vi "5.2.1.-SubVI Suavizado Gaussiano.vi"(6 "Capa de color":u32[][](array[numeric]), 7 "Sigma":dbl, 9 "T":dbl) -> (1 "Array out":i32[][](array[numeric]), 2 "J":i32[][](array[numeric]), 3 "h":dbl[][](array[numeric]))   [LabVIEW 2020]
panel:
  # "Visión Artificial - Reconocimiento de Bordes - Suavizado Filtro Gaussiano\nDiego Cervantes Rodríguez\ndicer0.com"
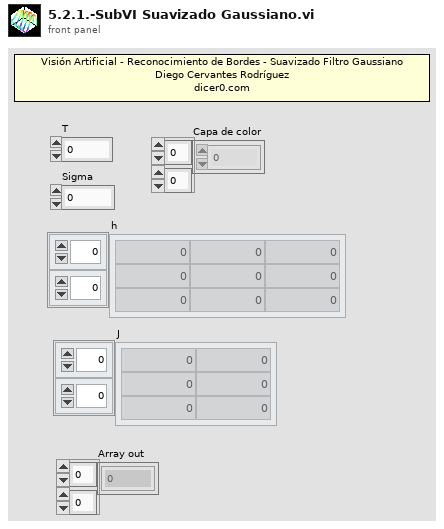
[diagram p1: front panel]
types:
  T1 = typedef "NI_Matrix.lvlib/RealMatrix.ctl" = dbl[][]
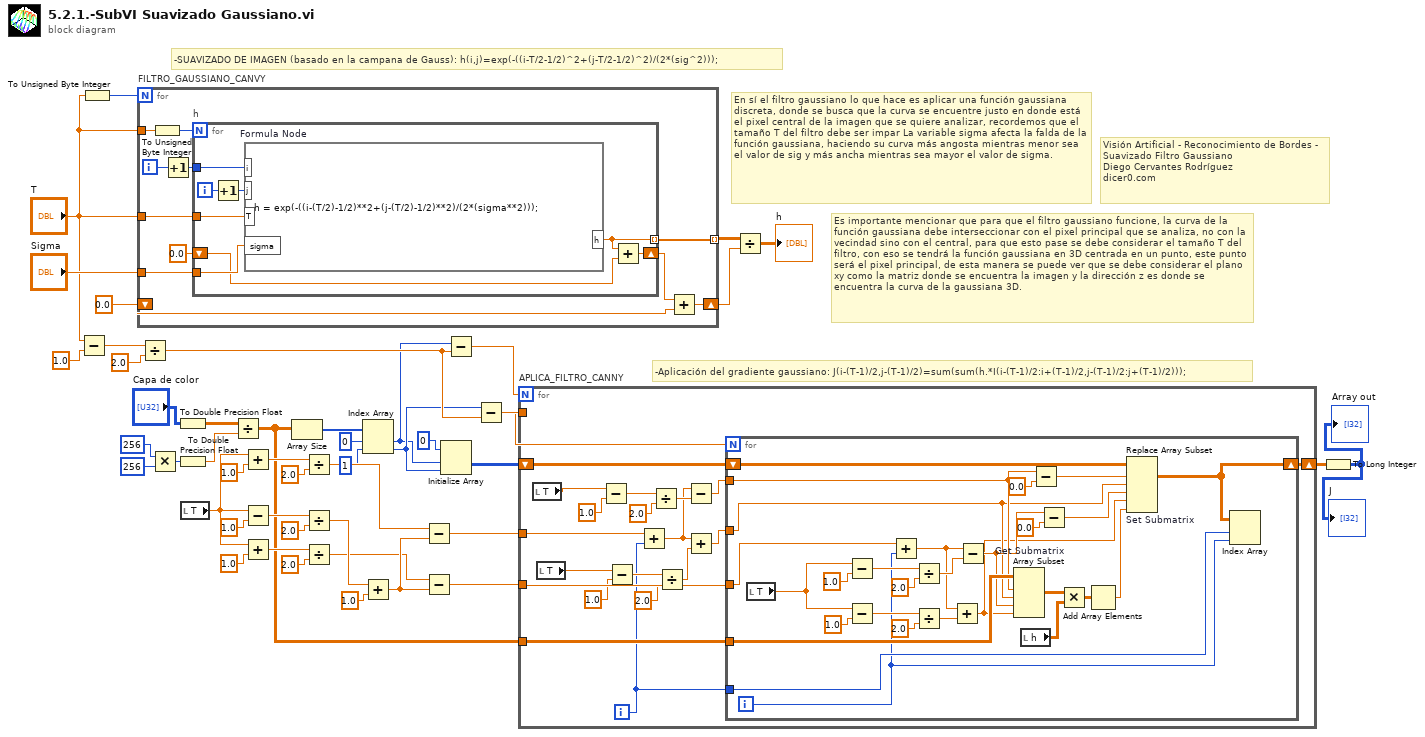
[diagram p0: block diagram]
diagram:
  # "Visión Artificial - Reconocimiento de Bordes - Suavizado Filtro Gaussiano\nDiego Cervantes Rodríguez\ndicer0.com"
  # "-Aplicación del gradiente gaussiano: J(i-(T-1)/2,j-(T-1)/2)=sum(sum(h.*I(i-(T-1)/2:i+(T-1)/2,j-(T-1)/2:j+(T-1)/2)));"
  # "Es importante mencionar que para que el filtro gaussiano funcione, la curva de la función gaussiana debe interseccionar con el pixel principal que se analiza, no con la vecindad sino con el central, para que esto pase se debe considerar el tamaño T del filtro, con eso se tendrá la función gaussiana en 3D centrada en un punto, este punto será el pixel principal, de esta manera se puede ver que se debe considerar el plano xy como la matriz donde se encuentra la imagen y la dirección z es donde se encuentra la curva de la gaussiana 3D."
  # "En sí el filtro gaussiano lo que hace es aplicar una función gaussiana discreta, donde se busca que la curva se encuentre justo en donde está el pixel central de la imagen que se quiere analizar, recordemos que el tamaño T del filtro debe ser impar La variable sigma afecta la falda de la función gaussiana, haciendo su curva más angosta mientras menor sea el valor de sig y más ancha mientras sea mayor el valor de sigma."
  # "-SUAVIZADO DE IMAGEN (basado en la campana de Gauss): h(i,j)=exp(-((i-T/2-1/2)^2+(j-T/2-1/2)^2)/(2*(sig^2)));"
  n1 = Subtract(x="T", y=1.0) -> (x-y=w20:dbl)
  n2 = To Unsigned Byte Integer(number="T") -> (unsigned 8bit integer=w9:u8)
  n3 = for "FILTRO_GAUSSIANO_CANVY" {
    N: w9 -> [_]
    tunnel: "T" -> [w47]
    tunnel: "T" -> [w57]
    tunnel: "Sigma" -> [w56]
    shift-right: [w53] -> w13
    shift-left: 0.0 ("h") -> [w51]
    tunnel: [w54] -> w12 mode=indexing
    i -> [w50]
    n4 = To Unsigned Byte Integer(number=w47) -> (unsigned 8bit integer=w48:u8)
    n5 = Increment(x=w50) -> (x+1=w49:i32)
    n6 = for "h" {
      N: w48 -> [_]
      tunnel: w57 -> [w65]
      tunnel: w56 -> [w64]
      tunnel: w49 -> [w63]
      shift-right: [w61] -> w52
      shift-left: 0.0 ("h") -> [w62]
      tunnel: [w60] -> w54 mode=indexing
      i -> [w59]
      n7 = Increment(x=w59) -> (x+1=w58:i32)
      n8 = formula code="h = exp(-((i-(T/2)-1/2)**2+(j-(T/2)-1/2)**2)/(2*(sigma**2)));"("T"=w65, "sigma"=w64, "i"=w63, "j"=w58) -> ("h"=w60:dbl)
      n9 = Add(x=w60, y=w62) -> (x+y=w61:dbl)
    }
    n10 = Add(x=w52, y=w51) -> (x+y=w53:dbl)
  }
  n11 = Divide(x=w20, y=2.0) -> (x/y=w23:dbl)
  n12 = Multiply(x=256, y=256) -> (x*y=w45:i32)
  n13 = To Double Precision Float(number="Capa de color") -> (double precision float=w43:dbl[][])
  n14 = To Double Precision Float(number=w45) -> (double precision float=w46:dbl)
  n15 = local read "T"() -> (w4:dbl)
  n16 = Divide(x=w43, y=w46) -> (x/y=w24:dbl[][])
  n17 = Add(x=w4, y=1.0) -> (x+y=w26:dbl)
  n18 = Subtract(x=w4, y=1.0) -> (x-y=w38:dbl)
  n19 = Add(x=w4, y=1.0) -> (x+y=w32:dbl)
  n20 = Array Size(array=w24) -> (size(s)=w16:i32[])
  n21 = Divide(x=w26, y=2.0) -> (x/y=w28:dbl)
  n22 = Divide(x=w38, y=2.0) -> (x/y=w40:dbl)
  n23 = Divide(x=w32, y=2.0) -> (x/y=w30:dbl)
  n24 = Index Array "Index Array"(array=w16, index #1=0 ("index"), index #2=1 ("index")) -> (element #1=w1:i32, element #2=w2:i32)
  n25 = Add(x=w40, y=1.0) -> (x+y=w42:dbl)
  n26 = Subtract(x=w28, y=w42) -> (x-y=w29:dbl)
  n27 = Subtract(x=w30, y=w42) -> (x-y=w34:dbl)
  n28 = Initialize Array "Initialize Array"(0 ("element"), w1, w2) -> (w36:i32[][])
  n29 = Subtract(x=w1, y=w23) -> (x-y=w3:dbl)
  n30 = Subtract(x=w2, y=w23) -> (x-y=w22:dbl)
  n31 = for "APLICA_FILTRO_CANNY" {
    N: w3 -> [_]
    tunnel: w22 -> [w85]
    tunnel: w24 -> [w84]
    tunnel: w29 -> [w83]
    tunnel: w34 -> [w82]
    shift-right: [w75] -> w6
    shift-left: w36 -> [w76]
    i -> [w66]
    n32 = local read "T"() -> (w68:dbl)
    n33 = local read "T"() -> (w67:dbl)
    n34 = Subtract(x=w68, y=1.0) -> (x-y=w81:dbl)
    n35 = Subtract(x=w67, y=1.0) -> (x-y=w73:dbl)
    n36 = Add(x=w83, y=w66) -> (x+y=w70:dbl)
    n37 = Divide(x=w81, y=2.0) -> (x/y=w78:dbl)
    n38 = Divide(x=w73, y=2.0) -> (x/y=w74:dbl)
    n39 = Subtract(x=w70, y=w78) -> (x-y=w77:dbl)
    n40 = Add(x=w70, y=w74) -> (x+y=w69:dbl)
    n41 = for {
      N: w85 -> [_]
      tunnel: w84 -> [w104]
      tunnel: w82 -> [w113]
      tunnel: w77 -> [w103]
      shift-right: [w93] -> w75
      shift-left: w76 -> [w95]
      tunnel: w66 -> [w107]
      tunnel: w69 -> [w90]
      i -> [w86]
      n42 = local read "T"() -> (w88:dbl)
      n43 = Subtract(x=w88, y=1.0) -> (x-y=w112:dbl)
      n44 = Subtract(x=w88, y=1.0) -> (x-y=w99:dbl)
      n45 = Add(x=w113, y=w86) -> (x+y=w96:dbl)
      n46 = Divide(x=w112, y=2.0) -> (x/y=w109:dbl)
      n47 = Divide(x=w99, y=2.0) -> (x/y=w100:dbl)
      n48 = Add(x=w96, y=w100) -> (x+y=w89:dbl)
      n49 = Subtract(x=w96, y=w109) -> (x-y=w102:dbl)
      n50 = Array Subset "Get Submatrix"(array=w104, index (row)=w103, length (row)=w90, index (col)=w102, length (col)=w89) -> (w101:dbl[][])
      n51 = local read "h"() -> (w87:dbl[][])
      n52 = Subtract(x=w103, y=0.0 ("x")) -> (x-y=w92:dbl)
      n53 = Subtract(x=w102, y=0.0 ("x")) -> (x-y=w91:dbl)
      n54 = Multiply ("Multiply.vi")(x=w101, y=w87) -> (x*y=w108:dbl[][])
      n55 = Add Array Elements(numeric array=w108) -> (sum=w94:dbl)
      n56 = Replace Array Subset "Set Submatrix"(array=w95, new element=w94, index (dim 0)=w92, index (dim 1)=w90, index (dim 2)=w91, index (dim 3)=w89) -> (w93:T1)
      n57 = Index Array "Index Array"(array=w93, index (row)=w107, index (col)=w86) -> ()  [unwired: 1 out]
    }
  }
  n58 = Divide(x=w12, y=w13) -> (x/y=→"h":dbl[][])
  n59 = To Long Integer(number=w6) -> (32bit integer=→"J" →"Array out":i32[][])
